vi "Remove Inputs with no Paired Output.vi"(8 "error in (no error)":errorcluster, 9 "Paired Module Output Channels":refnum<class "TBM channel.lvclass">[](array[class]), 10 "engine configuration in":refnum<class "engine configuration.lvclass">, 11 "E2E configuration in":refnum<class "E2E Tag Exchange configuration.lvclass">) -> (0 "error out":errorcluster, 2 "engine configuration out":refnum<class "engine configuration.lvclass">, 3 "E2E configuration out":refnum<class "E2E Tag Exchange configuration.lvclass">)   [LabVIEW 2015, in "E2E Tag Exchange editor node.lvclass"]
uses:
  E2E Tag Exchange editor node.lvclass
  <vilib>/NI/Tag Bus Module Framework/channel/TBM channel.lvclass
  <vilib>/NI/Module Execution Interface/Engine Configuration/engine configuration.lvclass
  module/configuration/E2E Tag Exchange configuration.lvclass
  <vilib>/NI/Tag Bus Module Framework/channel/channel classification.ctl
  <vilib>/NI/Tag Bus Module Framework/channel/TBM channel.lvclass/TBM channel.ctl
  <vilib>/NI/Configuration Framework/serializable configuration/NISE_CEF_serializable configuration.lvclass/NISE_CEF_serializable configuration.ctl
  <vilib>/Utility/LVClass/Get LV Class Name.vi
  <vilib>/NI/Configuration Framework/error generator/NISE_error generator.vi
  <vilib>/NI/Configuration Framework/serializable configuration/NISE_CEF_serializable configuration.lvclass
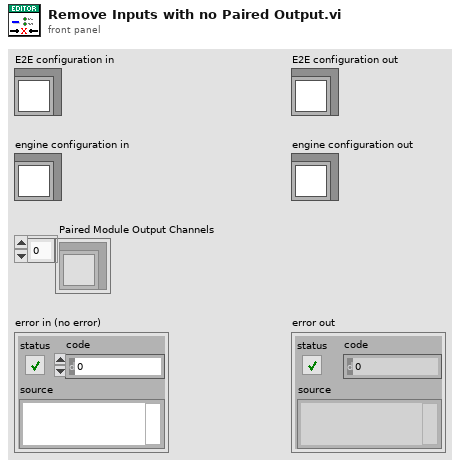
[diagram p1: front panel]
types:
  T1 = typedef "TBM channel.lvclass/channel classification.ctl" = enum16{"input data", "output data", "processing parameter", "processing result"}
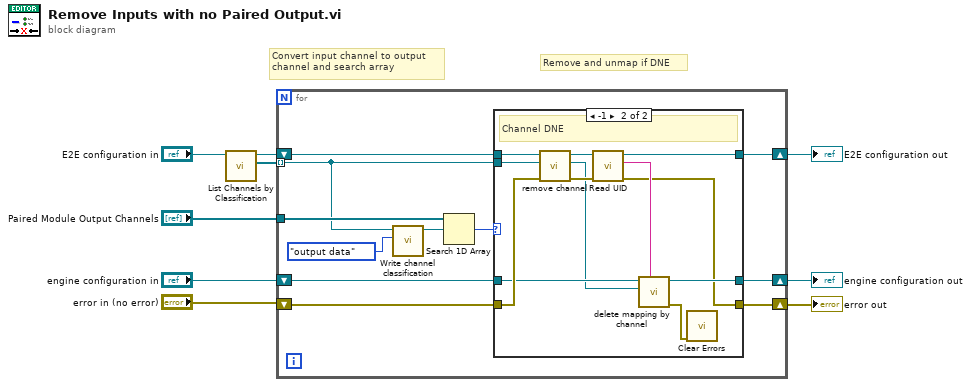
[diagram p0: block diagram]
diagram:
  # "Remove and unmap if DNE"
  # "Convert input channel to output\nchannel and search array"
  n1 = call "List Channels by Classification.vi"("E2E configuration in"="E2E configuration in") -> ("Input Channels"=w6:refnum<class "TBM channel.lvclass">[], "E2E configuration out"=w7:refnum<class "E2E Tag Exchange configuration.lvclass">)  [unwired: 8 in, 1 out]
  n2 = for {
    tunnel: "Paired Module Output Channels" -> [w13]
    tunnel: w6 -> [w10] mode=indexing
    shift-right: [w16] -> w2
    shift-left: "engine configuration in" -> [w18]
    shift-right: [w17] -> w1
    shift-left: w7 -> [w19]
    shift-right: [w15] -> w3
    shift-left: "error in (no error)" -> [w14]
    n3 = call <vilib>:"Write channel classification.vi"("channel classification"=channel_classification."output data", "channel in"=w10) -> ("channel out"=w12:refnum<class "TBM channel.lvclass">)  [unwired: 8 in, 1 out]
    n4 = Search 1D Array(1D array=w13, element=w12) -> (index of element=w11:i32)  [unwired: 1 in]
    n5 = case shown="-1" w11 {
      tunnel: w19 -> [w22 w35]
      tunnel: w18 -> [w21 w27]
      tunnel: [w22 w31] -> w17
      tunnel: [w21 w29] -> w16
      tunnel: [w23 w26] -> w15
      tunnel: w14 -> [w23 w34]
      tunnel: w10 -> [_ w33]
      frame Default {
        # "Channel Exists"
      }
      frame -1 {
        # "Channel DNE"
        n6 = call "remove channel.vi"("error in (no error)"=w34, "channel"=w33, "E2E configuration in"=w35) -> ("error out"=w30:errorcluster, "removed channel"=w24:refnum<class "TBM channel.lvclass">, "E2E configuration out"=w32:refnum<class "E2E Tag Exchange configuration.lvclass">)  [unwired: 6 in]
        n7 = call <vilib>:"Read UID.vi"("error in"=w30, "configuration in"=w32) -> ("error out"=w26:errorcluster, "instance id"=w28:string, "configuration out"=w31:refnum<class "E2E Tag Exchange configuration.lvclass">)  [unwired: 7 in]
        n8 = call <vilib>:"delete mapping by channel.vi"("owner ID"=w28, "channel"=w24, "engine configuration in"=w27) -> ("error out"=w25:errorcluster, "engine configuration out"=w29:refnum<class "engine configuration.lvclass">)  [unwired: 7 in]
        n9 = call <vilib>:"Clear Errors.vi"("error in (no error)"=w25) -> ()  [unwired: 5 in, 2 out]
      }
    }
  }
  "E2E configuration out" <- w1
  "engine configuration out" <- w2
  "error out" <- w3
